vi "Begin.vi"(8 "error in":errorcluster) -> (0 "error out":errorcluster)   [LabVIEW 2015]
doc: "Called before other user functions, this VI can be used to open I/O refnums, load in file data, and do general program initialization. Notice that the <B>error out</B> terminal is simply used for data flow. Wiring it to other structures or subVIs ensures that this VI runs first."
uses:
  <vilib>/Rock Robotics/WPI/DriverStation/WPI_DriverStationRobotMode2.ctl
  <vilib>/Rock Robotics/WPI/Joystick/WPI_JoystickDeviceEnum.ctl
  <vilib>/Rock Robotics/SystemInterfaces/DIO/FPGA_DIOChannel.ctl
  Robot Global Data.vi
  <vilib>/Rock Robotics/Network Tables/NT Write String Array.vi
  <vilib>/Rock Robotics/WPI/Counter/WPI_CounterDigitalInputToDigitalSource.vi
  <vilib>/Rock Robotics/WPI/Switch/WPI_SwitchOpenLimit.vi
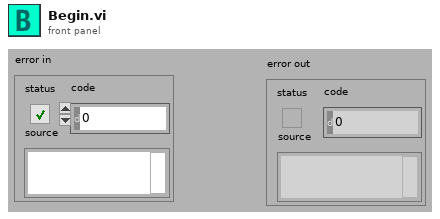
[diagram p1: front panel]
types:
  T1 = typedef "FPGA_DIOChannel.ctl" = enum8{"DIO 0", "DIO 1", "DIO 2", "DIO 3", "DIO 4", "DIO 5", "DIO 6", "DIO 7", "DIO 8", "DIO 9", "DIO MXP 0", "DIO MXP 1", "DIO MXP 2", "DIO MXP 3", "DIO MXP 4", "DIO MXP 5", "DIO MXP 6", "DIO MXP 7", "DIO MXP 8", "DIO MXP 9", "DIO MXP 10", "DIO MXP 11", "DIO MXP 12", "DIO MXP 13", "DIO MXP 14", "DIO MXP 15", "Invalid"}
  T2 = typedef "WPI_JoystickDeviceEnum.ctl" = enum16{"USB 0", "USB 1", "USB 2", "USB 3", "USB 4", "USB 5"}
  T3 = typedef "WPI_DriverStationRobotMode2.ctl" = enum16{"Autonomous Disabled", "Autonomous Enabled", "Teleop Disabled", "Teleop Enabled", "Disconnected", "Finish", "Test Disabled", "Test Enabled", "Emergency Stopped"}
  T4 = typedef "WPI_JoystickDevRef.ctl" = cluster{"Device":T2}
  T5 = typedef "WPI_DigitalInputDevRef.ctl" = cluster{"DevStatus":errorcluster, "DIO Channel":T1}
  T6 = typedef "FPGA_CounterEncoderSourceConvertionLVSourceType.ctl" = cluster{"DevStatus":errorcluster, "AnalogTriggerMode?":bool, "DigitalMode":cluster{"DIO Channel":T7}, "AnalogTriggerMode":cluster{"AnalogTriggerIndex":T8, "OutputType":T9}}
  T7 = typedef "FPGA_DIODigitalSourceChannel.ctl" = enum8{"DIO 0", "DIO 1", "DIO 2", "DIO 3", "DIO 4", "DIO 5", "DIO 6", "DIO 7", "DIO 8", "DIO 9", "DIO MXP 0", "DIO MXP 1", "DIO MXP 2", "DIO MXP 3", "DIO MXP 4", "DIO MXP 5", "DIO MXP 6", "DIO MXP 7", "DIO MXP 8", "DIO MXP 9", "DIO MXP 10", "DIO MXP 11", "DIO MXP 12", "DIO MXP 13", "DIO MXP 14", "DIO MXP 15", "Disabled"}
  T8 = typedef "FPGA_AnalogTriggerIndex.ctl" = enum8{"Trig 0", "Trig 1", "Trig 2", "Trig 3", "Trig 4", "Trig 5", "Trig 6", "Trig 7", "Invalid"}
  T9 = typedef "FPGA_AnalogTriggerOutType.ctl" = enum16{"InWindow", "TriggerState", "Rising", "Falling"}
  T10 = typedef "WPI_EncoderDevRef.ctl" = cluster{"DevStatus":errorcluster, "EncoderIndex":T11, "CounterIndex":T12, "DistancePerCount":dbl, "Decoding Type":T13}
  T11 = typedef "FPGA_EncoderIdx.ctl" = enum8{"Enc 0", "Enc 1", "Enc 2", "Enc 3", "Enc 4", "Enc 5", "Enc 6", "Enc 7", "Invalid"}
  T12 = typedef "FPGA_CounterCtrSystemIndex.ctl" = enum8{"Ctr 0", "Ctr 1", "Ctr 2", "Ctr 3", "Ctr 4", "Ctr 5", "Ctr 6", "Ctr 7", "Invalid"}
  T13 = typedef "WPI_EncoderType.ctl" = enum16{"1x", "2x", "4x"}
  T14 = typedef "WPI_SwitchDevRef.ctl" = cluster{"DevStatus":errorcluster, "DIO Channel":T1, "CntIndex":T12, "Normally Closed":bool}
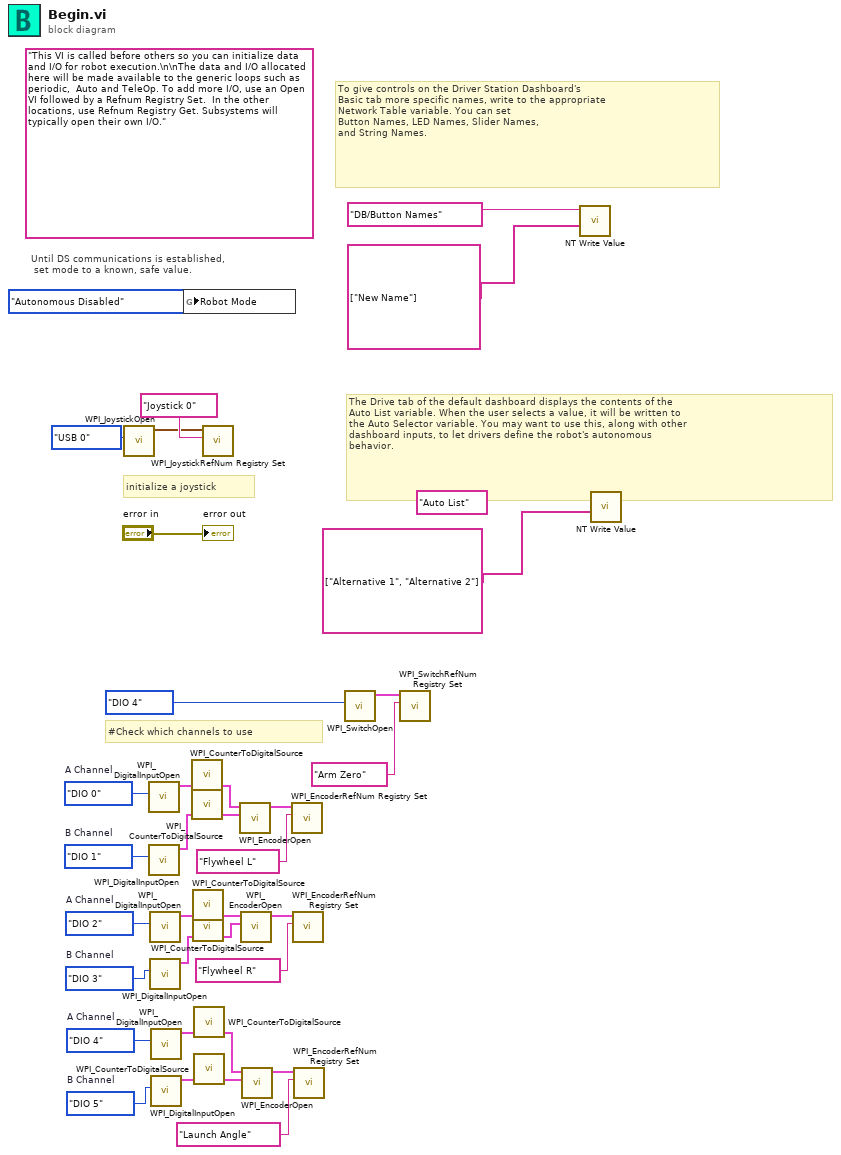
[diagram p0: block diagram]
diagram:
  w8 = FPGA_DIOChannel."DIO 3"  # B Channel
  w7 = FPGA_DIOChannel."DIO 2"  # A Channel
  w9 = FPGA_DIOChannel."DIO 5"  # B Channel
  w19 = FPGA_DIOChannel."DIO 4"  # A Channel
  w27 = FPGA_DIOChannel."DIO 1"  # B Channel
  w26 = FPGA_DIOChannel."DIO 0"  # A Channel
  (unwired) "This VI is called before others so you can initialize data and I/O for robot execution.\n\nThe data and I/O allocated here will be made available to the generic loops such as periodic,  Auto and TeleOp. To add more I/O, use an Open VI followed by a Refnum Registry Set.  In the other locations, use Refnum Registry Get. Subsystems will typically open their own I/O."
  # "#Check which channels to use"
  # "The Drive tab of the default dashboard displays the contents of the\nAuto List variable. When the user selects a value, it will be written to\nthe Auto Selector variable. You may want to use this, along with other\ndashboard inputs, to let drivers define the robot's autonomous\nbehavior."
  # "To give controls on the Driver Station Dashboard's\nBasic tab more specific names, write to the appropriate\nNetwork Table variable. You can set\nButton Names, LED Names, Slider Names,\nand String Names."
  # "initialize a joystick"
  # "Until DS communications is established,\n set mode to a known, safe value."
  n1 = call <vilib>:"WPI_JoystickOpen.vi"("JoystickDevice"=WPI_JoystickDeviceEnum."USB 0") -> ("JoystickDevRef"=w34:T4)  [unwired: 10 in]
  n2 = call <vilib>:"WPI_DigitalInputOpen.vi"("DIO Channel"=w26) -> ("DigitalInputDevRef"=w23:T5)  [unwired: 1 in, 9 out]
  n3 = call <vilib>:"WPI_DigitalInputOpen.vi"("DIO Channel"=w27) -> ("DigitalInputDevRef"=w24:T5)  [unwired: 1 in, 9 out]
  n4 = call <vilib>:"WPI_DigitalInputOpen.vi"("DIO Channel"=w7) -> ("DigitalInputDevRef"=w4:T5)  [unwired: 1 in, 9 out]
  n5 = call <vilib>:"WPI_DigitalInputOpen.vi"("DIO Channel"=w8) -> ("DigitalInputDevRef"=w5:T5)  [unwired: 1 in, 9 out]
  n6 = call <vilib>:"WPI_DigitalInputOpen.vi"("DIO Channel"=w19) -> ("DigitalInputDevRef"=w16:T5)  [unwired: 1 in, 9 out]
  n7 = call <vilib>:"WPI_DigitalInputOpen.vi"("DIO Channel"=w9) -> ("DigitalInputDevRef"=w17:T5)  [unwired: 1 in, 9 out]
  n8 = global write "Robot Global Data.vi" "Robot Mode"(WPI_DriverStationRobotMode2."Autonomous Disabled" ("Robot Mode")) -> ()
  n9 = call-poly <vilib>:"WPI_CounterToDigitalSource.vi"("DigitalInputDevRef"=w23) -> ("Digital Source"=w22:T6)  [unwired: 6 out]
  n10 = call-poly <vilib>:"WPI_CounterToDigitalSource.vi"("DigitalInputDevRef"=w24) -> ("Digital Source"=w25:T6)  [unwired: 6 out]
  n11 = call-poly <vilib>:"WPI_CounterToDigitalSource.vi"("DigitalInputDevRef"=w4) -> ("Digital Source"=w3:T6)  [unwired: 6 out]
  n12 = call-poly <vilib>:"WPI_CounterToDigitalSource.vi"("DigitalInputDevRef"=w5) -> ("Digital Source"=w6:T6)  [unwired: 6 out]
  n13 = call-poly <vilib>:"WPI_CounterToDigitalSource.vi"("DigitalInputDevRef"=w16) -> ("Digital Source"=w15:T6)  [unwired: 6 out]
  n14 = call-poly <vilib>:"WPI_CounterToDigitalSource.vi"("DigitalInputDevRef"=w17) -> ("Digital Source"=w18:T6)  [unwired: 6 out]
  n15 = call <vilib>:"WPI_JoystickRefNum Registry Set.vi"("refnum name"="Joystick 0", "JoystickDevRef"=w34) -> ()  [unwired: 8 in, 2 out]
  n16 = call <vilib>:"WPI_EncoderOpen.vi"("BSource"=w25, "ASource"=w22) -> ("EncoderDevRef"=w21:T10)  [unwired: 6 in, 3 out]
  n17 = call <vilib>:"WPI_EncoderOpen.vi"("BSource"=w6, "ASource"=w3) -> ("EncoderDevRef"=w2:T10)  [unwired: 6 in, 3 out]
  n18 = call <vilib>:"WPI_EncoderOpen.vi"("BSource"=w18, "ASource"=w15) -> ("EncoderDevRef"=w14:T10)  [unwired: 6 in, 3 out]
  n19 = call <vilib>:"WPI_EncoderRefNum Registry Set.vi"("refnum name"="Flywheel L", "EncoderDevRef"=w21) -> ()  [unwired: 8 in, 2 out]
  n20 = call <vilib>:"WPI_EncoderRefNum Registry Set.vi"("refnum name"="Flywheel R", "EncoderDevRef"=w2) -> ()  [unwired: 8 in, 2 out]
  n21 = call <vilib>:"WPI_EncoderRefNum Registry Set.vi"("refnum name"="Launch Angle", "EncoderDevRef"=w14) -> ()  [unwired: 8 in, 2 out]
  n22 = call-poly <vilib>:"WPI_SwitchOpen.vi"("DIO Channel"=FPGA_DIOChannel."DIO 4") -> ("SwitchDevRef"=w12:T14)  [unwired: 9 in, 1 out]
  n23 = call <vilib>:"WPI_SwitchRefNum Registry Set.vi"("refnum name"="Arm Zero", "SwitchDevRef"=w12) -> ()  [unwired: 8 in, 2 out]
  n24 = call-poly <vilib>:"NT Write Value.vi"("String Array"=string[] ["New Name"], "Name"="DB/Button Names") -> ()  [unwired: 9 in, 1 out]
  n25 = call-poly <vilib>:"NT Write Value.vi"("String Array"=string[] ["Alternative 1", "Alternative 2"], "Name"="Auto List") -> ()  [unwired: 9 in, 1 out]
  "error out" <- "error in"
